vi "Get Process from Map.vi"(8 "error in (no error)":errorcluster, 10 "Process Name":string, 11 "Application In":refnum<class "Application.lvclass">) -> (0 "error out":errorcluster, 2 "Process":refnum<class "Process.lvclass">, 3 "Application Out":refnum<class "Application.lvclass">)   [LabVIEW 2020, in "Application.lvclass"]
uses:
  Application.lvclass
  Process/Process.lvclass
  Application.lvclass/Application.ctl
  <vilib>/Utility/error.llb/Error Cluster From Error Code.vi
  <vilib>/ErrorRing/Error Ring.xnode
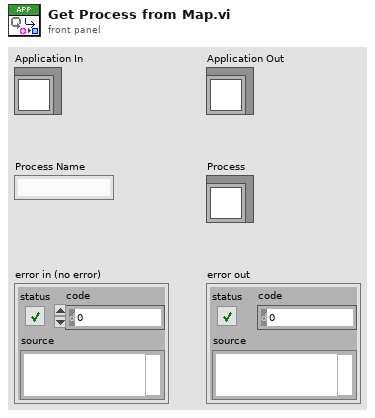
[diagram p1: front panel]
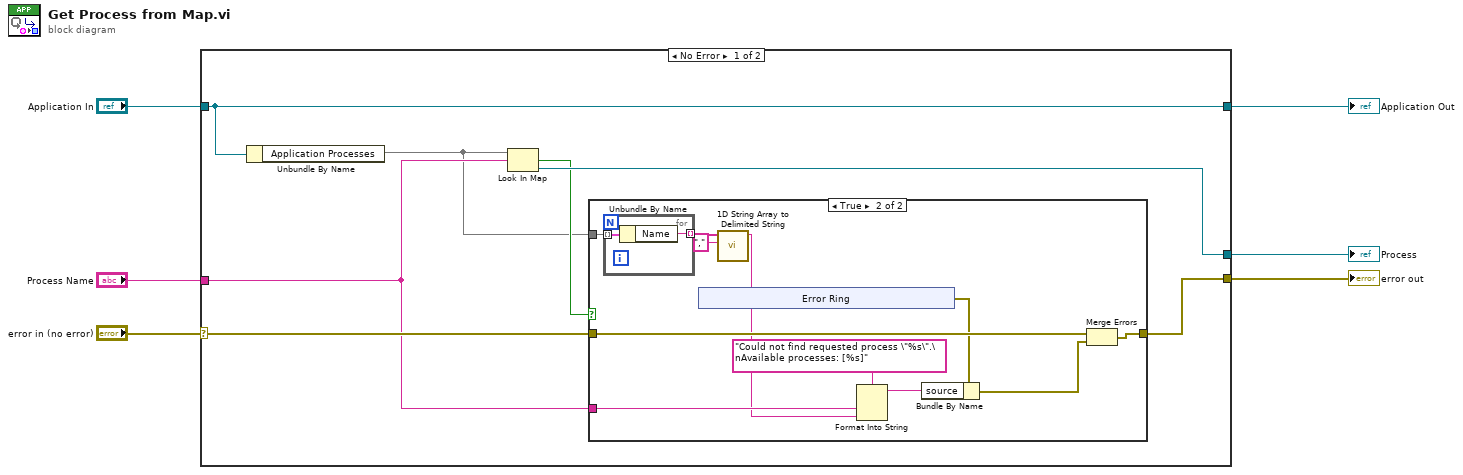
[diagram p0: block diagram]
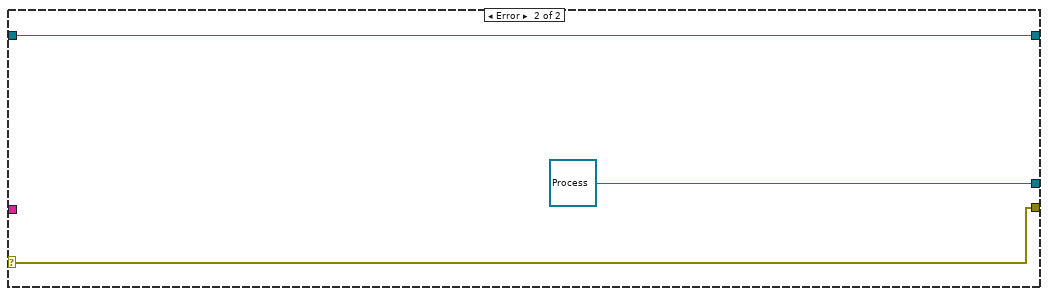
[diagram p3: hidden frame]
diagram:
  n1 = case shown="No Error" "error in (no error)" {
    selector: "error in (no error)" -> [w10 w34]
    tunnel: [w13 refnum<class "Process.lvclass"> refnum ("Process")] -> w6
    tunnel: [w12 w34] -> w5
    tunnel: [w11 w33] -> w4
    tunnel: "Application In" -> [w11 w33]
    tunnel: "Process Name" -> [w9 _]
    frame No Error {
      n2 = Unbundle By Name(w11) -> ("Application Processes"=w7:map{string, refnum<class "Process.lvclass">})
      n3 = Look In Map(map=w7, key=w9) -> (key not found?=w8:bool, value=w13:refnum<class "Process.lvclass">)  [unwired: 1 in]
      n4 = case shown="True" w8 {
        tunnel: [w14 w25] -> w12
        tunnel: w10 -> [w14 w24]
        tunnel: w9 -> [_ w20]
        tunnel: w7 -> [_ w18]
        frame False {
        }
        frame True {
          n5 = for {
            tunnel: w18 -> [w27] mode=indexing
            tunnel: [w26] -> w17 mode=indexing
            n6 = Unbundle By Name(w27) -> ("Name"=w26:string)
          }
          n7 = xnode "Error Ring"() -> ("error out"=w23:errorcluster)
          n8 = call <vilib>:"1D String Array to Delimited String.vi"("delimiter"=",", "string array"=w17) -> ("delimited string"=w15:string)  [unwired: 9 in]
          n9 = Format Into String(format string="Could not find requested process \"%s\".\nAvailable processes: [%s]", w20, w15) -> (resulting string=w19:string)  [unwired: 2 in, 1 out]
          n10 = Bundle By Name(cluster=w23, "source"=w19) -> (w22:errorcluster)
          n11 = Merge Errors(w24, w22) -> (w25:errorcluster)
        }
      }
    }
    frame Error {
    }
  }
  "Process" <- w6
  "error out" <- w5
  "Application Out" <- w4
